vi "Video File Frame Read.vi"(8 "error in (no error)":errorcluster, 10 "Image Dst":T1, 11 "Realsense Cam File Wrapper in":refnum<class "Realsense Cam File Wrapper.lvclass">) -> (0 "error out":errorcluster, 2 "Video Frame out":refnum<class "Video Frame.lvclass">, 3 "Realsense Cam File Wrapper out":refnum<class "Realsense Cam File Wrapper.lvclass">, 4 "Playback Finished?":bool, 6 "Looped?":bool)   [LabVIEW 2018, in "Realsense Cam File Wrapper.lvclass"]
uses:
  Realsense Cam File Wrapper.lvclass
  C:/Users/aaron.jencks/Documents/GitHub/emerson_seed_object_detection/LabVIEW/Projects/Paul's Video Viewer/Classes/Video File/Video File.lvclass
  <vilib>/vision/Image Controls.llb/IMAQ Image.ctl
  Video Frame/Video Frame.lvclass
  Video File/Video File.lvclass/Video File.ctl
  Realsense Cam File Wrapper.lvclass/Realsense Cam File Wrapper.ctl
  Video File/Read Frame Data.vi
  ROIed Video Frame/ROIed Video Frame.lvclass
  C:/Users/aaron.jencks/Documents/GitHub/emerson_seed_object_detection/LabVIEW/Projects/Paul's Video Viewer/Classes/Video Frame/Video Frame.lvclass
  Realsense Cam/Realsense Cam.lvclass
  Video File/Video File.lvclass
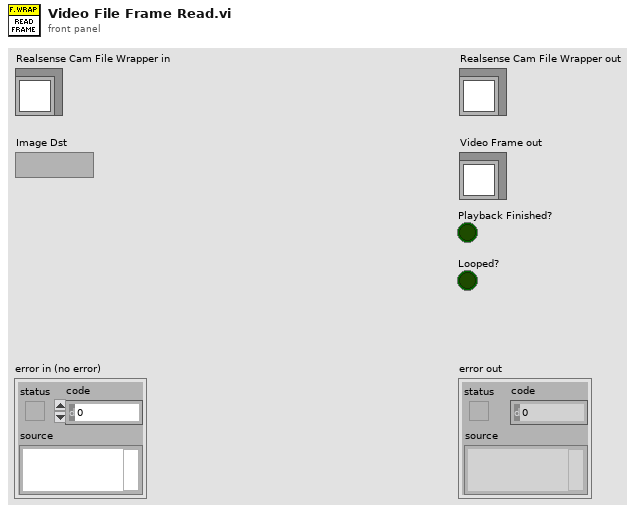
[diagram p1: front panel]
types:
  T1 = typedef "IMAQ Image.ctl" = refnum<image>
  T2 = typedef "Realsense Cam.lvclass/Cam Profiles STYP.ctl" = cluster{"IR":cluster{"Left":cluster{"Normal":T3, "Unrectified":T3}, "Right":cluster{"Normal":T3, "Unrectified":T3}}, "Color":cluster{"Color Left":T3, "RGB Ext.":T3}, "Depth":T3}
  T3 = typedef "Realsense Cam.lvclass/Stream STYP.ctl" = cluster{"Strings":string[], "Intrinsics":cluster{"width":i32, "height":i32, "fps":i32, "Profile":u64, "ppx":sgl, "ppy":sgl, "fx":sgl, "fy":sgl, "model":u32}[], "Current Data":T4}
  T4 = typedef "Realsense Cam.lvclass/Stream Frame Data STYP.ctl" = cluster{"Depths":sgl[][], "Bytes":u8[], "16-Bit IR":u16[], "Height":i32, "Width":i32}
  T5 = typedef "Image Type" = u32
  T6 = cluster{"Width":u32, "Height":u32, "Frames Per Second":u32, "Codec":string, "Has Data":bool}
  T7 = cluster{"Global Rectangle":i32[], "Contours":cluster{"Contour Type":u32, "ROI Type":u32, "Points":i32[]}[]}
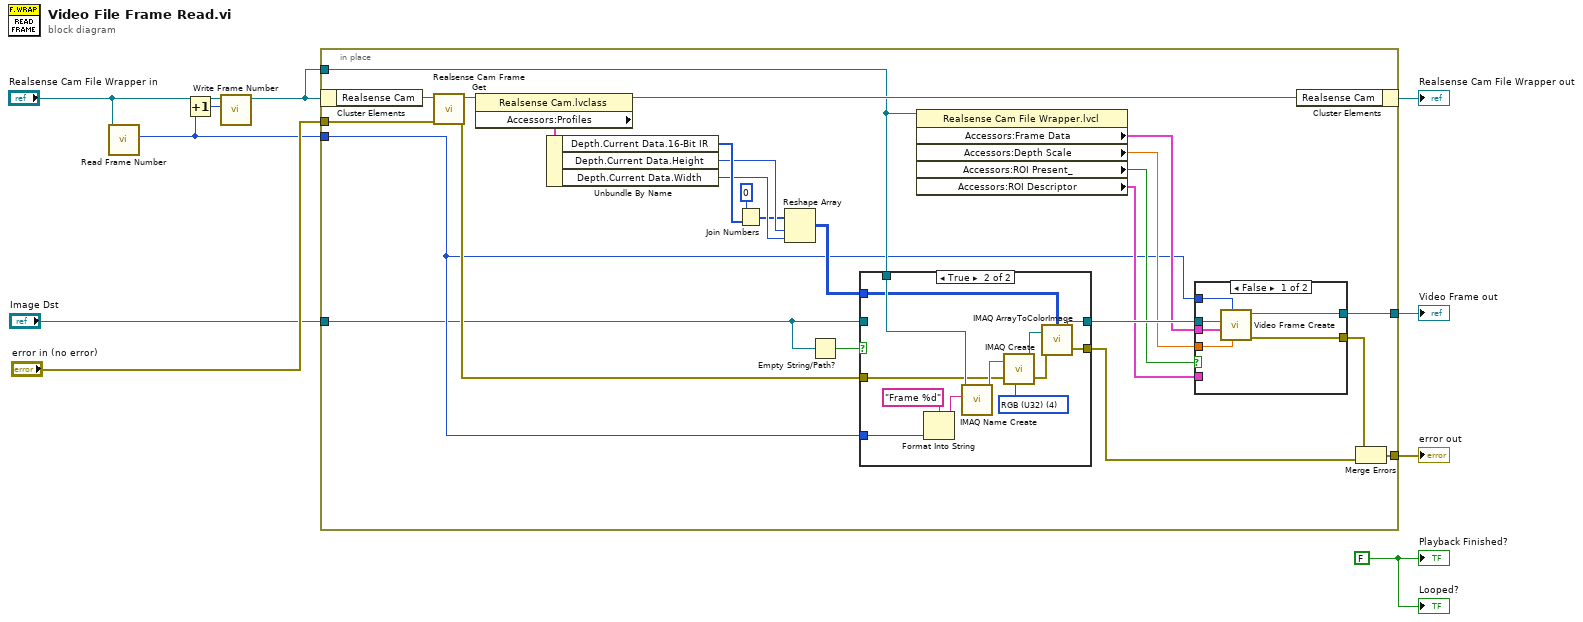
[diagram p0: block diagram]
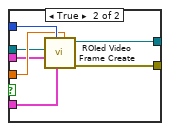
[diagram p2: hidden frame]
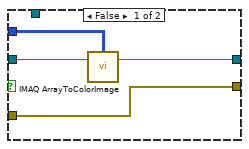
[diagram p3: hidden frame]
diagram:
  w1 = FALSE
  n1 = call "Read Frame Number.vi"("Video File in"="Realsense Cam File Wrapper in") -> ("Frame Number"=w6:u32)  [unwired: 8 in, 2 out]
  n2 = Increment(x=w6) -> (x+1=w7:u32)
  n3 = call "Write Frame Number.vi"("Frame Number"=w7, "Video File in"="Realsense Cam File Wrapper in") -> ("Video File out"=w4:refnum<class "Realsense Cam File Wrapper.lvclass">)  [unwired: 8 in, 1 out]
  n4 = in-place {
    in-place-border: "error in (no error)" -> [w34]
    in-place-border: "Image Dst" -> [w11]
    in-place-border: w4 -> [w23]
    in-place-border: w6 -> [w17]
    in-place-border: [w16] -> w3
    in-place-border: [w13] -> w2
    n5 = in-place-cluster #1(w4) -> ("Realsense Cam"=w35:refnum<class "Realsense Cam.lvclass">)
    n6 = call-dynamic "Realsense Cam Frame Get.vi"("error in (no error)"=w34, "Realsense Cam in"=w35) -> ("error out"=w24:errorcluster, "Realsense Cam out"=w33:refnum<class "Realsense Cam.lvclass">)  [unwired: 8 in]
    n7 = property class="Realsense Cam.lvclass"(reference=w33) -> (reference out=w31:refnum<class "Realsense Cam.lvclass">, "Accessors:Profiles"=w32:T2)  [unwired: 1 in, 1 out]
    n8 = Unbundle By Name(w32) -> ("Depth.Current Data.16-Bit IR"=w29:u16[], "Depth.Current Data.Height"=w28:i32, "Depth.Current Data.Width"=w27:i32)
    n9 = Join Numbers(hi=u16 0, lo=w29) -> ((hi.lo)=w26:u32[])
    n10 = Reshape Array(w26, w28, w27) -> (w25:u32[][])
    n11 = Empty String/Path?(string/path=w11) -> (empty?=w12:bool)
    n12 = case shown="True" w12 {
      tunnel: w11 -> [w51 _]
      tunnel: [w50 w58] -> w22
      tunnel: w25 -> [w52 w57]
      tunnel: [w49 w59] -> w14
      tunnel: w23 -> [_ w61]
      tunnel: w24 -> [w49 w60]
      tunnel: w17 -> [_ w54]
      frame False {
        n13 = call "IMAQ ArrayToColorImage"("Image Pixels (U32)"=w52, "Image"=w51) -> ("Image Out"=w50:T1)  [unwired: 3 in, 1 out]
      }
      frame True {
        w53 = T5 4 items=["Grayscale (U8)", "Grayscale (I16)", "Grayscale (SGL)", "Complex (CSG)", "RGB (U32)", "HSL (U32)", "RGB (U64)", "Grayscale (U16)"] ("Image Type")
        n14 = Format Into String(format string="Frame %d", w54) -> (resulting string=w63:string)  [unwired: 2 in, 1 out]
        n15 = call "IMAQ Name Create.vi"("Name (\"\")"=w63, "Video File in"=w61) -> ("Name Out"=w64:string)  [unwired: 7 in, 2 out]
        n16 = call "IMAQ Create"("Image Name"=w64, "Image Type"=w53, "error in (no error)"=w60) -> ("New Image"=w56:T1, "error out"=w55:errorcluster)  [unwired: 2 in]
        n17 = call "IMAQ ArrayToColorImage"("Image Pixels (U32)"=w57, "Image"=w56, "error in (no error)"=w55) -> ("Image Out"=w58:T1, "error out"=w59:errorcluster)  [unwired: 2 in]
      }
    }
    n18 = property class="Realsense Cam File Wrapper.lvcl"(reference=w23) -> ("Accessors:Frame Data"=w18:T6, "Accessors:Depth Scale"=w19:dbl, "Accessors:ROI Present_"=w20:bool, "Accessors:ROI Descriptor"=w21:T7)  [unwired: 1 in, 2 out]
    n19 = case shown="False" w20 {
      tunnel: w22 -> [w41 w46]
      tunnel: w17 -> [w40 w48]
      tunnel: w18 -> [w39 w45]
      tunnel: w19 -> [w38 w47]
      tunnel: [w37 w43] -> w16
      tunnel: w21 -> [_ w44]
      tunnel: [w36 w42] -> w15
      frame False {
        n20 = call "Video Frame Create.vi"("Depth Scale"=w38, "Frame Number"=w40, "Frame Data"=w39, "Image Dst"=w41) -> ("error out"=w36:errorcluster, "Video Frame out"=w37:refnum<class "Video Frame.lvclass">)  [unwired: 6 in]
      }
      frame True {
        n21 = call "ROIed Video Frame Create.vi"("Depth Scale"=w47, "ROI Descriptor"=w44, "Frame Number"=w48, "Frame Data"=w45, "Image Dst"=w46) -> ("error out"=w42:errorcluster, "ROIed Video Frame out"=w43:refnum<class "ROIed Video Frame.lvclass">)  [unwired: 5 in]
      }
    }
    n22 = in-place-cluster #1("Realsense Cam"=w31) -> (→"Realsense Cam File Wrapper out":refnum<class "Realsense Cam File Wrapper.lvclass">)
    n23 = Merge Errors(w15, w14) -> (w13:errorcluster)
  }
  "error out" <- w2
  "Video Frame out" <- w3
  "Playback Finished?" <- w1
  "Looped?" <- w1
